vi "lab1.2.vi"() -> ()   [LabVIEW 2021]
uses:
  <vilib>/express/express analysis/Spectral/Block/exnSpectralBlock spectral measurements peak poly.vi
  <vilib>/express/express analysis/Spectral/Block/exnSpectralBlock spectral measurements peak WFM.vi
  <vilib>/measure/maspectr.llb/FFT Spectrum (Mag-Phase) for N Chan.vi
  <vilib>/measure/maspectr.llb/FFT Spectrum (Mag-Phase) for 1 Chan.vi
  <vilib>/express/express analysis/Spectral/XNode/ExpressSpectralMeasurementsBlockNode.xnode
  <vilib>/measure/NI_MAPro.lvlib
  <vilib>/measure/NI_MABase.lvlib
panel:
  out "Waveform Graph TEST":waveform(dbl)(graph)
  out "Waveform Graph TEST":cluster{"f0":dbl, "df":dbl, "magnitude":dbl[]}(graph)
  in  "Upper sıde":i32
  in  "Lower sıde":i32
  in  "frequency":dbl=10.0 format="%0.2p"
  in  "sampling info":cluster{"Fs":dbl, "#s":dbl}={"Fs"=1000.0, "#s"=1000.0} {"Fs" format="%.2p"}
  out "Waveform Graph 5":cluster{"f0":dbl, "df":dbl, "magnitude":dbl[]}(graph)
  out "Waveform Graph 4":cluster{"f0":dbl, "df":dbl, "magnitude":dbl[]}[](graph)
  out "Waveform Graph with zero padding 2":waveform(dbl)(graph)
  out "output array 2":dbl[](array[numeric])
  out "initialized array 2":dbl[](array[numeric])
  out "Waveform Graph 3":dynamicdata(graph)
  out "Waveform Graph  with zero  padding":cluster{"f0":dbl, "df":dbl, "magnitude":dbl[]}(graph)
  out "Waveform Graph with zero padding":waveform(dbl)(graph)
  out "output array":dbl[](array[numeric])
  out "initialized array":dbl[](array[numeric])
  out "Waveform Graph 2":cluster{"f0":dbl, "df":dbl, "magnitude":dbl[]}(graph)
  out "Waveform Graph":waveform(dbl)(graph)
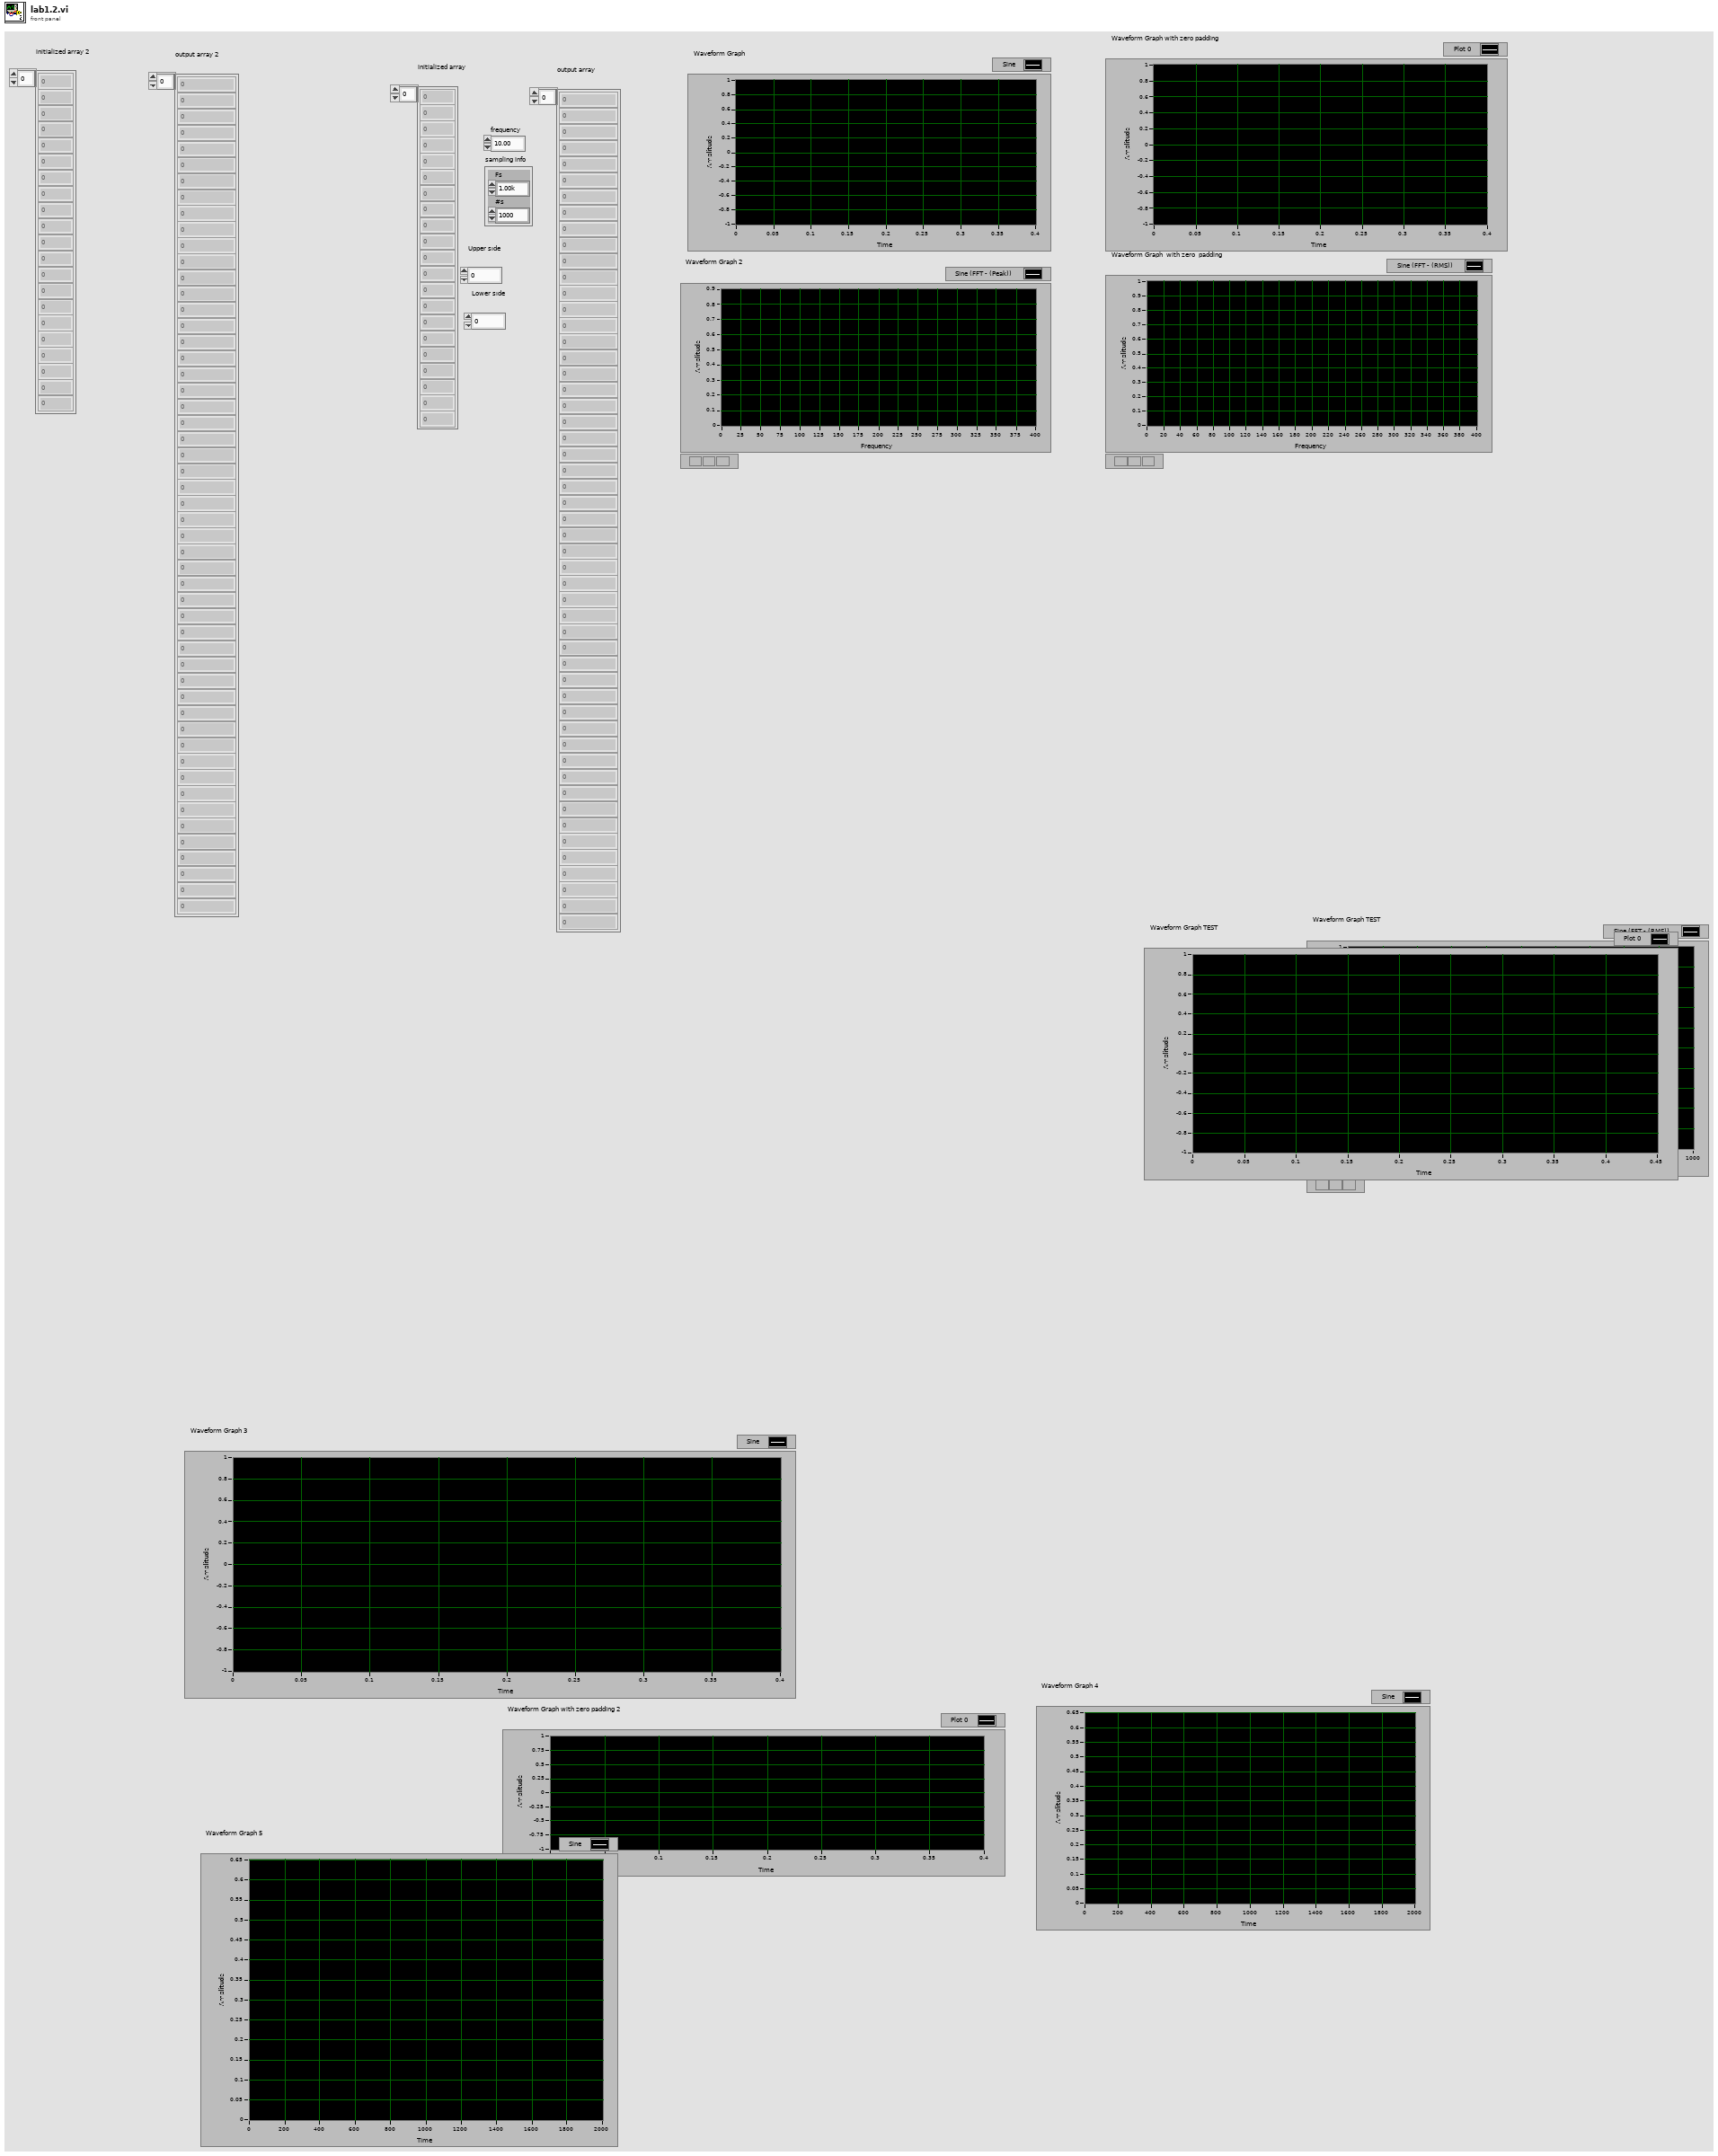
[diagram p1: front panel]
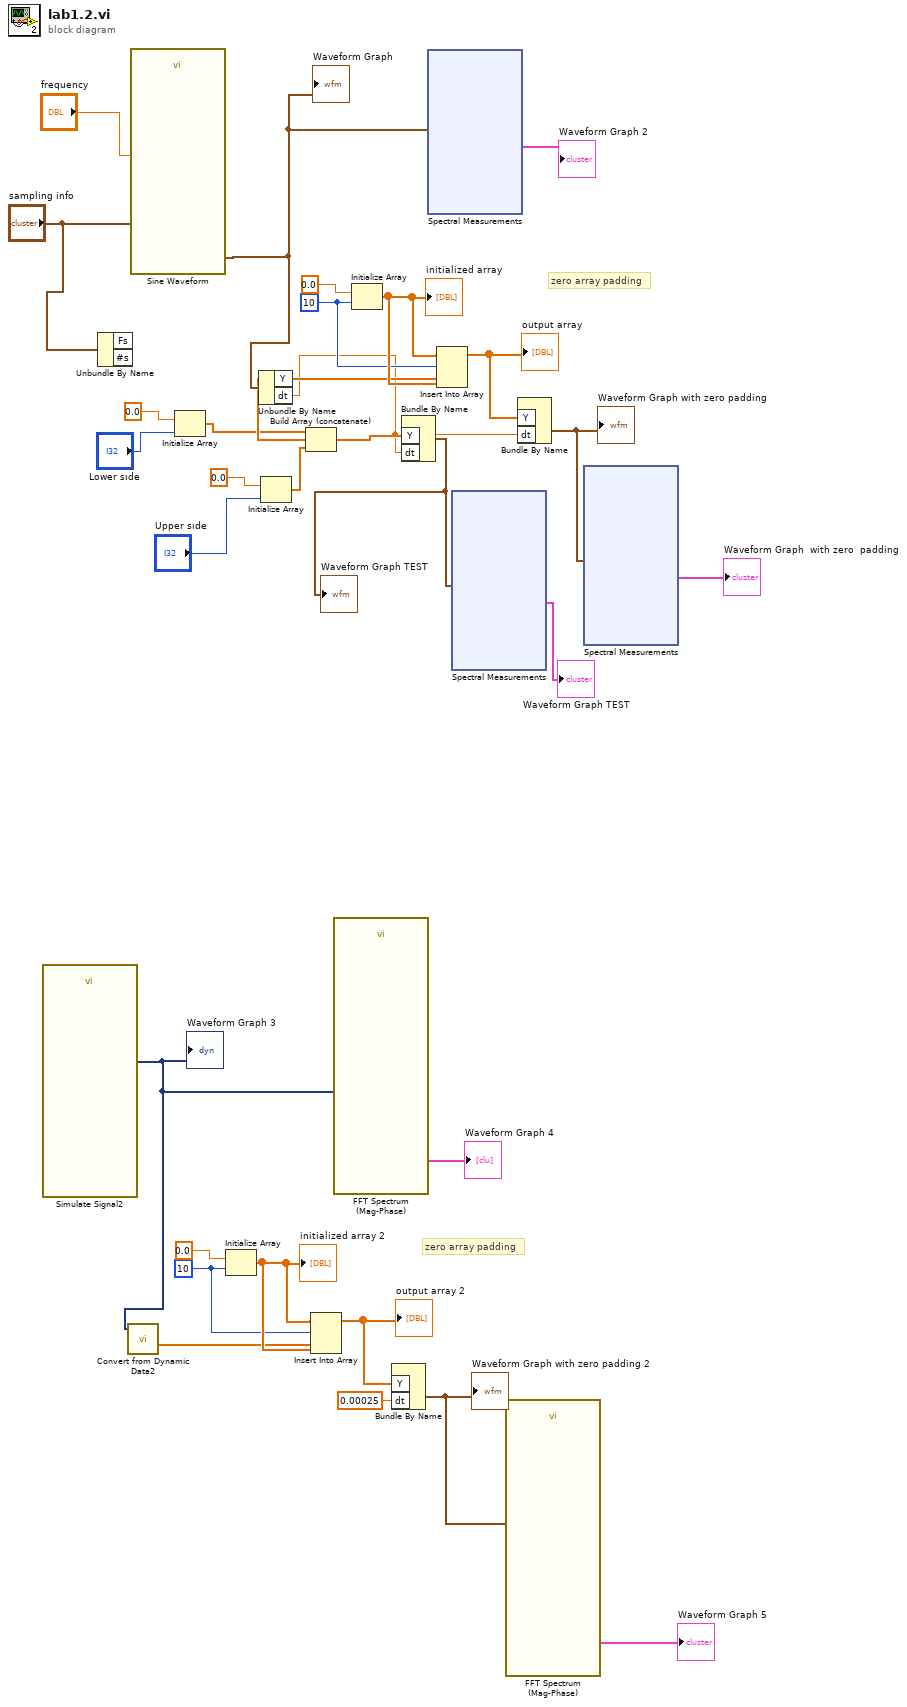
[diagram p0: block diagram]
diagram:
  w19 = 10 ("dimension size")
  w26 = 10 ("dimension size")
  # "zero array padding"
  # "zero array padding"
  n1 = call "Simulate Signal2"() -> ("Sine"=w18:dynamicdata)  [unwired: 14 in, 1 out]
  "Waveform Graph 3" <- w18
  n2 = Unbundle By Name("sampling info") -> ()  [unwired: 2 out]
  n3 = call "Convert from Dynamic Data2"("Dynamic Data Type"=w18) -> ("Array"=w20:dbl[])  [unwired: 3 in]
  n4 = call <vilib>:"Sine Waveform.vi"("sampling info"="sampling info", "frequency"="frequency") -> ("signal out"=w12:waveform(dbl))  [unwired: 8 in, 1 out]
  "Waveform Graph" <- w12
  n5 = Initialize Array(0.0 ("element"), "Lower sıde") -> (w9:dbl[])
  n6 = Initialize Array(0.0 ("element"), w19) -> (w23:dbl[])
  "initialized array 2" <- w23
  n7 = Unbundle By Name(w12) -> ("Y"=w11:dbl[], "dt"=w3:dbl)
  n8 = Initialize Array(0.0 ("element"), "Upper sıde") -> (w4:dbl[])
  n9 = Build Array (concatenate)(w9, w11, w4) -> (w7:dbl[])
  n10 = Insert Into Array(array=w23, index=w19, new element #1=w20, new element #2=w23) -> (w22:dbl[])
  "output array 2" <- w22
  n11 = call-poly <vilib>:"FFT Spectrum (Mag-Phase).vi"("time signals"=w18) -> ("magnitudes"=→"Waveform Graph 4":cluster{"f0":dbl, "df":dbl, "magnitude":dbl[]}[])  [unwired: 6 in, 4 out]
  n12 = Initialize Array(0.0 ("element"), w26) -> (w29:dbl[])
  "initialized array" <- w29
  n13 = Bundle By Name("Y"=w22, "dt"=0.00025) -> (w15:waveform(dbl))  [unwired: 1 in]
  "Waveform Graph with zero padding 2" <- w15
  n14 = Bundle By Name("Y"=w7, "dt"=w3) -> (w1:waveform(dbl))  [unwired: 1 in]
  "Waveform Graph TEST" <- w1
  n15 = xnode "Spectral Measurements"("Signals"=w12) -> ("FFT - (Peak)"=→"Waveform Graph 2":cluster{"f0":dbl, "df":dbl, "magnitude":dbl[]})  [unwired: 1 in, 2 out]
  n16 = Insert Into Array(array=w29, index=w26, new element #1=w11, new element #2=w29) -> (w28:dbl[])
  "output array" <- w28
  n17 = xnode "Spectral Measurements"("Signals"=w1) -> ("FFT - (Peak)"=→"Waveform Graph TEST":cluster{"f0":dbl, "df":dbl, "magnitude":dbl[]})  [unwired: 1 in, 2 out]
  n18 = call-poly <vilib>:"FFT Spectrum (Mag-Phase).vi"("time signal"=w15) -> ("magnitude"=→"Waveform Graph 5":cluster{"f0":dbl, "df":dbl, "magnitude":dbl[]})  [unwired: 6 in, 4 out]
  n19 = Bundle By Name("Y"=w28, "dt"=w3) -> (w27:waveform(dbl))  [unwired: 1 in]
  "Waveform Graph with zero padding" <- w27
  n20 = xnode "Spectral Measurements"("Signals"=w27) -> ("FFT - (Peak)"=→"Waveform Graph  with zero  padding":cluster{"f0":dbl, "df":dbl, "magnitude":dbl[]})  [unwired: 1 in, 2 out]
